vi "Start.vi"(8 "error in (no error)":errorcluster, 10 "mode (current)":u16(ring) items=["current mode", "internal", "external", "without amplifier"], 11 "Lotis in":refnum<class "PL Lotis TII LS.lvclass">) -> (0 "error out":errorcluster, 3 "Lotis out":refnum<class "PL Lotis TII LS.lvclass">)   [LabVIEW 2015, in "PL Lotis TII LS.lvclass"]
doc: "Starts generation."
uses:
  PL Lotis TII LS.lvclass
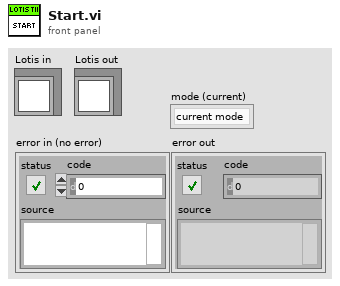
[diagram p1: front panel]
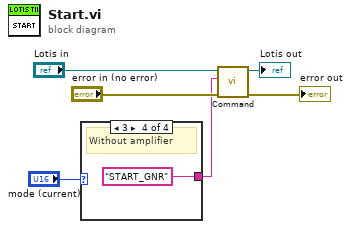
[diagram p0: block diagram]
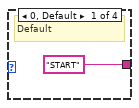
[diagram p2: hidden frame]
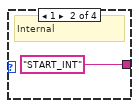
[diagram p3: hidden frame]
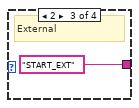
[diagram p4: hidden frame]
diagram:
  n1 = case shown="3" "mode (current)" {
    tunnel: ["START" ("command") "START_INT" ("command") "START_EXT" ("command") "START_GNR" ("command")] -> w1
    frame 0, Default {
      # "Default"
    }
    frame 1 {
      # "Internal"
    }
    frame 2 {
      # "External"
    }
    frame 3 {
      # "Without amplifier"
    }
  }
  n2 = call "Command.vi"("error in (no error)"="error in (no error)", "command"=w1, "Lotis in"="Lotis in") -> ("error out"=→"error out":errorcluster, "Lotis out"=→"Lotis out":refnum<class "PL Lotis TII LS.lvclass">)  [unwired: 6 in, 1 out]
